vi "Test CFG file.vi"() -> ()   [LabVIEW 2015]
uses:
  Hardware/LakeShore/Lake Shore Temperature Controller/LakeShore T Controller.lvclass
  <vilib>/Utility/config.llb/NI_LVConfig.lvlib
panel:
  in  "CFG File":path
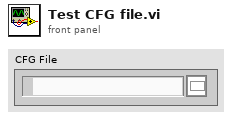
[diagram p1: front panel]
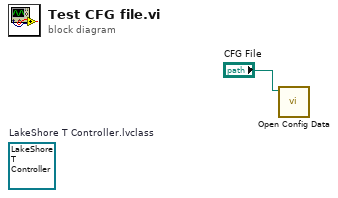
[diagram p0: block diagram]
diagram:
  (unwired) refnum<class "LakeShore T Controller.lvclass"> refnum  # LakeShore T Controller.lvclass
  n1 = call <vilib>:"Open Config Data.vi"("configuration file path"="CFG File") -> ()  [unwired: 8 in, 3 out]
